vi "Addition.vi"() -> ()   [LabVIEW 2018]
panel:
  in  "1":dbl
  out "3":dbl
  out "1":dbl
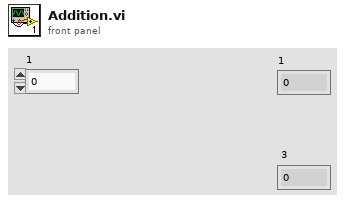
[diagram p1: front panel]
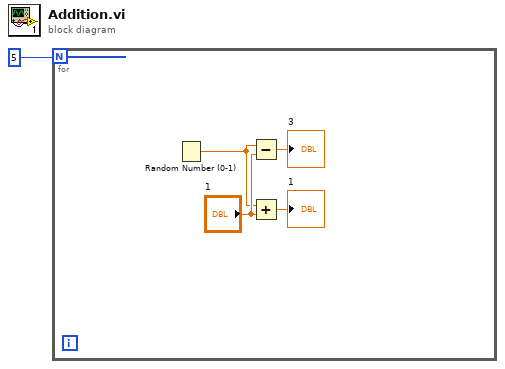
[diagram p0: block diagram]
diagram:
  n1 = for {
    N: 5 -> [_]
    n2 = Random Number (0-1)() -> (number: 0 to 1=w2:dbl)
    n3 = Subtract(x=w2, y="1") -> (x-y=→"3":dbl)
    n4 = Add(x=w2, y="1") -> (x+y=→"1":dbl)
  }
